vi "DCA Compute T-R2.vi"(1 "Measurement Values":T1) -> (0 "T-R2":dbl)   [LabVIEW 2011]
uses:
  TypeDefs/DCA Measurement Values.ctl
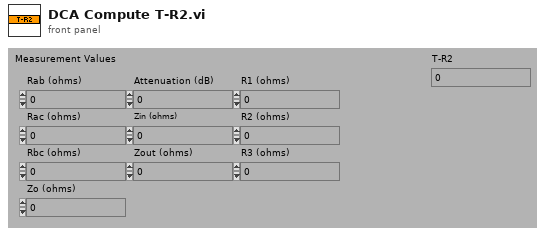
[diagram p1: front panel]
types:
  T1 = typedef "DCA Measurement Values.ctl" = cluster{"Rab (ohms)":dbl, "Rac (ohms)":dbl, "Rbc (ohms)":dbl, "Zo (ohms)":dbl, "Attenuation (dB)":dbl, "Zin (ohms)":dbl, "Zout (ohms)":dbl, "R1 (ohms)":dbl, "R2 (ohms)":dbl, "R3 (ohms)":dbl}
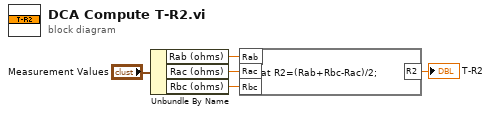
[diagram p0: block diagram]
diagram:
  n1 = Unbundle By Name("Measurement Values") -> ("Rab (ohms)"=w4:dbl, "Rac (ohms)"=w3:dbl, "Rbc (ohms)"=w2:dbl)
  n2 = formula code="float R2=(Rab+Rbc-Rac)/2;"("Rab"=w4, "Rac"=w3, "Rbc"=w2) -> ("R2"=→"T-R2":dbl)
